vi "main.vi"() -> ()   [LabVIEW 2018]
uses:
  <userlib>/ORI_DataSocketReader/DataSocket Tag Reader.lvclass
  ControlConfigMisura.ctl
  ControlConfigDI.ctl
panel:
  in  "Tab Control":enum32{"Valori", "Storico allarmi"}(tab)
  in  "Misure":i32(listbox)
  in  "fine":timestamp format="%<%Y-%m-%d %H:%M>T"
  in  "Inizio":timestamp format="%<%Y-%m-%d %H:%M>T"
  in  "Storico":i32(listbox)
  out "last":string
  in  "ack":bool
  out "Uscita digitale":bool
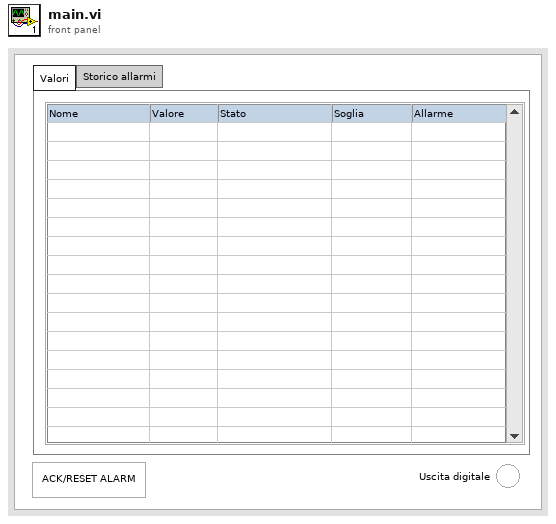
[diagram p1: front panel]
types:
  T1 = typedef "ControlConfigMisura.ctl" = cluster{"svVal":string, "svInvDig":T2[], "nome":string, "valore":dbl, "stato":i16, "soglia":dbl, "allarme":bool, "enable":bool}
  T2 = typedef "ControlConfigDI.ctl" = cluster{"sv":string, "na":bool, "valRaw":bool, "val":bool}
  T3 = typedef "ControlCfg.ctl" = cluster{"misure":T1[], "SVDO":string}
  T4 = typedef "LVPoint32TypeDef.ctl" = cluster{"Horizontal":i32, "Vertical":i32}
  T5 = typedef "LVRowAndColumnTypeDef.ctl" = cluster{"Row":i32, "Column":i32}
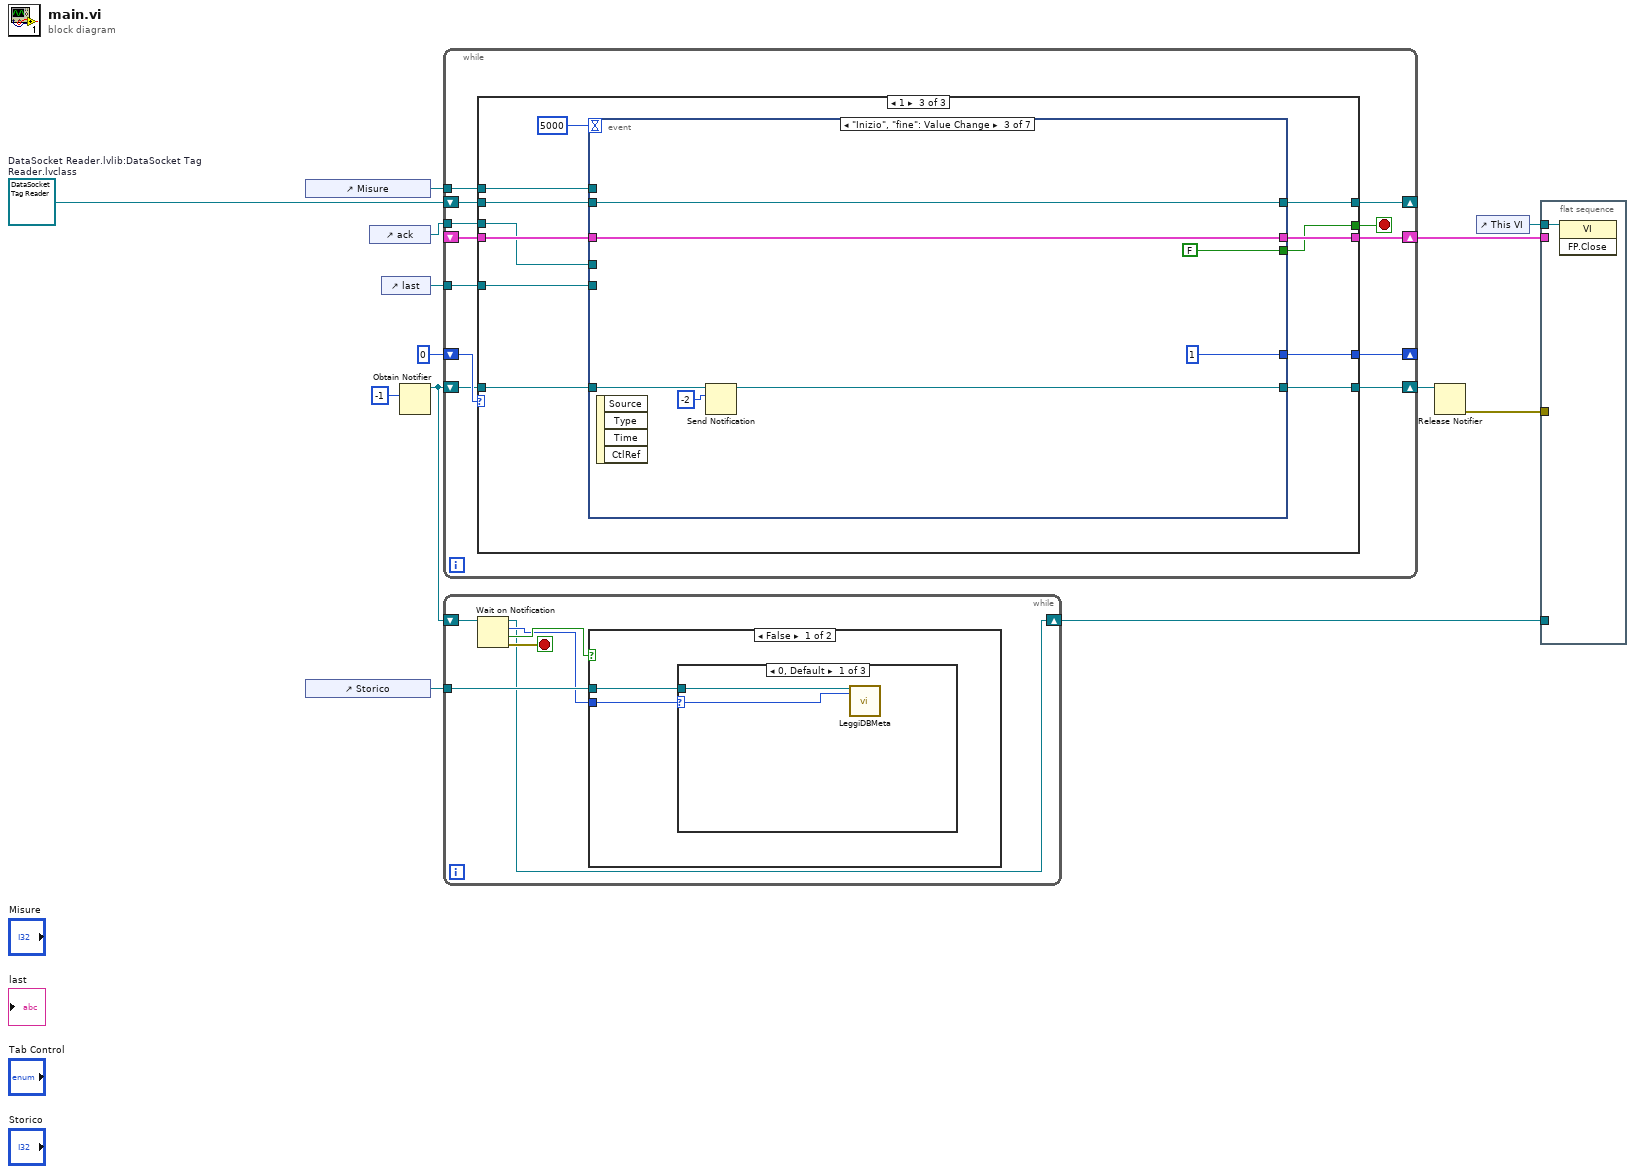
[diagram p0: block diagram]
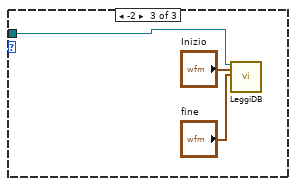
[diagram p3: hidden frame]
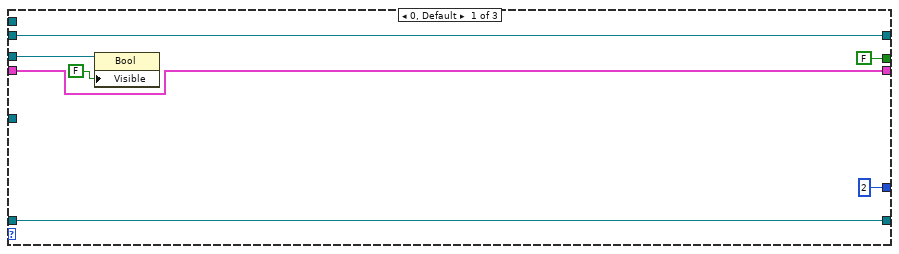
[diagram p5: hidden frame]
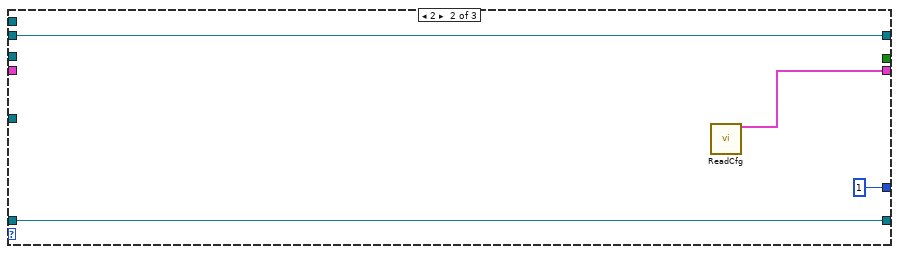
[diagram p6: hidden frame]
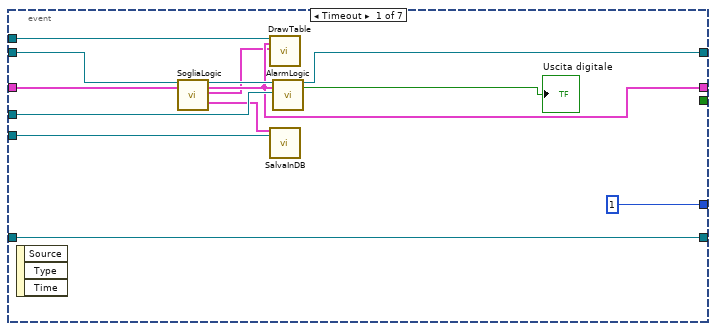
[diagram p7: hidden frame]
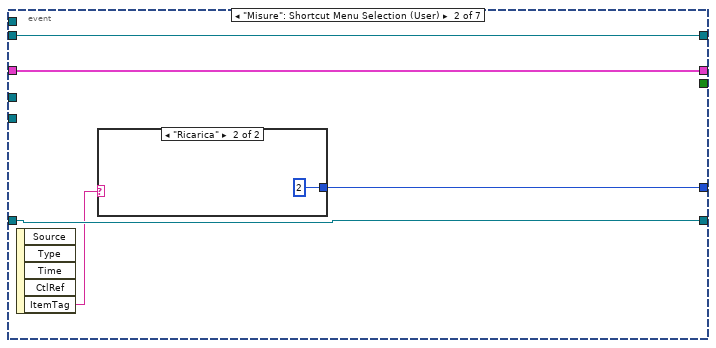
[diagram p8: hidden frame]
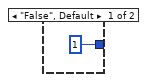
[diagram p9: hidden frame]
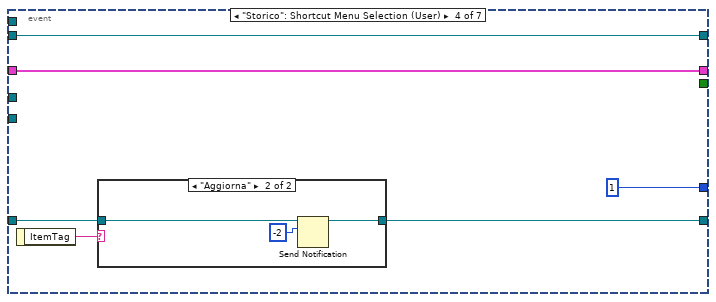
[diagram p10: hidden frame]
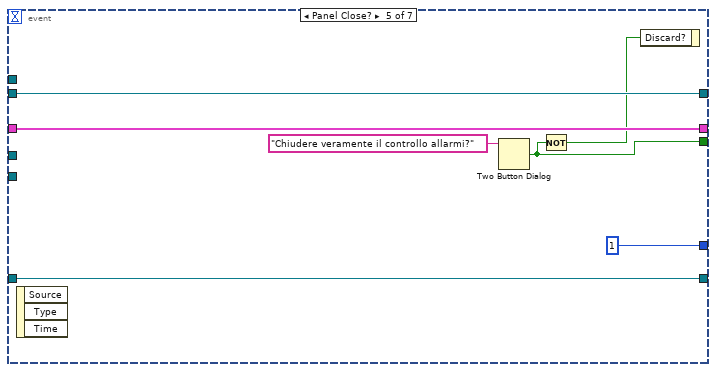
[diagram p12: hidden frame]
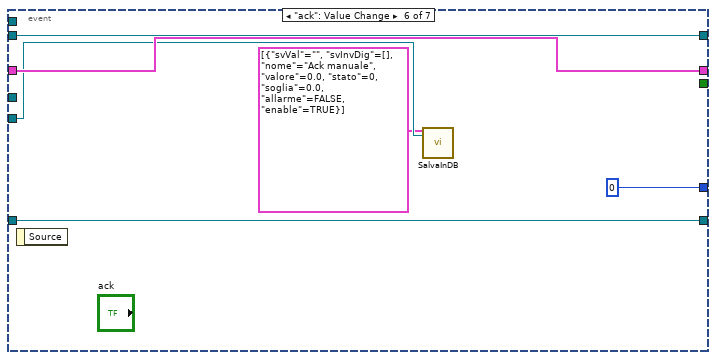
[diagram p13: hidden frame]
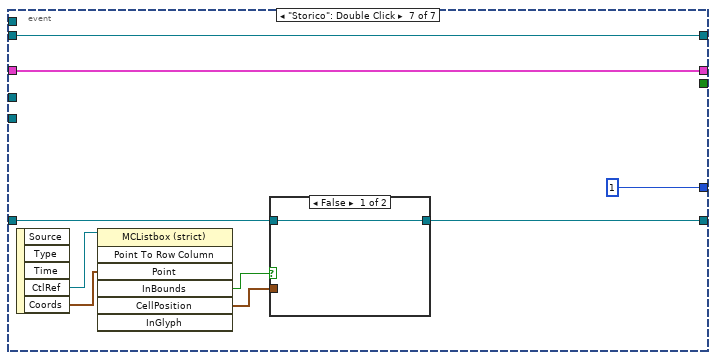
[diagram p14: hidden frame]
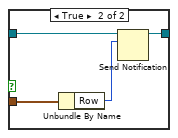
[diagram p15: hidden frame]
diagram:
  w12 = refnum<class "DataSocket Tag Reader.lvclass"> refnum  # DataSocket Reader.lvlib:DataSocket Tag Reader.lvclass
  n1 = control-ref of="Misure"() -> (w11:refnum<vi>)
  n2 = control-ref of="Storico"() -> (w5:refnum<vi>)
  n3 = control-ref of="ack"() -> (w10:refnum<vi>)
  n4 = control-ref of="last"() -> (w7:refnum<vi>)
  n5 = Obtain Notifier(notification data type=-1) -> (notifier out=w6:refnum<notifier>)  [unwired: 3 in, 2 out]
  n6 = while {
    shift-right: [w23] -> _
    shift-left: 0 -> [w25]
    shift-right: [w21] -> _
    shift-left: w12 -> [w22]
    shift-right: [w20] -> w8
    shift-left: _ -> [w19]
    tunnel: w11 -> [w18]
    tunnel: w10 -> [w17]
    tunnel: w7 -> [w16]
    shift-right: [w14] -> w4
    shift-left: w6 -> [w15]
    stop <- w24 stop-if-true
    n7 = case shown="1" w25 {
      tunnel: [FALSE _ w40] -> w24
      tunnel: [2 1 w47] -> w23
      tunnel: w22 -> [w30 w36 w46]
      tunnel: [w30 w36 w45] -> w21
      tunnel: [w26 w34 w43] -> w20
      tunnel: w19 -> [w26 _ w44]
      tunnel: w18 -> [_ _ w42]
      tunnel: w17 -> [w29 _ w41]
      tunnel: w16 -> [_ _ w39]
      tunnel: w15 -> [w28 w35 w38]
      tunnel: [w28 w35 w37] -> w14
      frame 0, Default {
        n8 = property class="Bool"(reference=w29, "Visible"=FALSE) -> ()  [unwired: 1 in, 2 out]
      }
      frame 2 {
        n9 = call "ReadCfg.vi"() -> ("data"=w34:T3)  [unwired: 19 in]
      }
      frame 1 {
        n10 = event shown="[2] \"Inizio\", \"fine\": Value Change" {
          selector: _ -> [_ _ _ _ _ _ _]
          dyn-events: _ -> [_ _ _ _ _ _ _]
          timeout: 5000 -> [_ _ _ _ _ _ _]
          tunnel: [1 w62 1 1 1 0 1] -> w47
          tunnel: w46 -> [w60 w64 w75 w81 w91 w96 w107]
          tunnel: [w55 w64 w75 w81 w91 w96 w107] -> w45
          tunnel: w44 -> [w59 w63 w72 w80 w90 w97 w106]
          tunnel: [w54 w63 w72 w80 w90 w97 w106] -> w43
          tunnel: w42 -> [w58 _ _ _ _ _ _]
          tunnel: w41 -> [w57 _ _ _ _ _ _]
          tunnel: [_ _ FALSE ("T button?") _ w88 _ _] -> w40
          tunnel: w39 -> [w50 _ _ _ _ w94 _]
          tunnel: w38 -> [w49 w66 w71 w77 w86 w95 w104]
          tunnel: [w49 w66 w70 w76 w86 w95 w103] -> w37
          event Timeout {
            n11 = event-data() -> ()  [unwired: 1 in, 3 out]
            n12 = call "SogliaLogic.vi"("DSR"=w60, "cfg"=w59) -> ("DSR out"=w56:refnum<class "DataSocket Tag Reader.lvclass">, "cfg out"=w54:T3, "Array"=w52:cluster{bool[], string[]}[], "CambiStato"=w51:T1[])  [unwired: 14 in]
            n13 = call "DrawTable.vi"("Table"=w58, "cfg"=w54, "Array"=w52) -> ()  [unwired: 17 in]
            n14 = call "SalvaInDB.vi"("CambiStato"=w51, "last"=w50) -> ()  [unwired: 18 in]
            n15 = call "AlarmLogic.vi"("DSR"=w56, "cfg"=w54, "ack"=w57) -> ("DSR out"=w55:refnum<class "DataSocket Tag Reader.lvclass">, "AllarmeSuDO"=→"Uscita digitale":bool)  [unwired: 15 in]
          }
          event "Misure": Shortcut Menu Selection (User) {
            n16 = event-data() -> ("ItemTag"=w65:string)  [unwired: 1 in, 4 out]
            n17 = case shown="\"Ricarica\"" w65 {
              tunnel: [1 2] -> w62
              frame "False", Default {
              }
              frame "Ricarica" {
              }
            }
          }
          event "Inizio", "fine": Value Change {
            n18 = event-data() -> ()  [unwired: 1 in, 4 out]
            n19 = Send Notification(notification=-2, notifier=w71) -> (notifier out=w70:refnum<notifier>)  [unwired: 1 in, 1 out]
          }
          event "Storico": Shortcut Menu Selection (User) {
            n20 = event-data() -> ("ItemTag"=w78:string)  [unwired: 1 in]
            n21 = case shown="\"Aggiorna\"" w78 {
              tunnel: w77 -> [w82 w85]
              tunnel: [w82 w84] -> w76
              frame "False", Default {
              }
              frame "Aggiorna" {
                n22 = Send Notification(notification=-2, notifier=w85) -> (notifier out=w84:refnum<notifier>)  [unwired: 1 in, 1 out]
              }
            }
          }
          event Panel Close? {
            n23 = event-data() -> ()  [unwired: 1 in, 3 out]
            n24 = Two Button Dialog(message="Chiudere veramente il controllo allarmi?") -> (T button?=w88:bool)  [unwired: 2 in]
            n25 = Not(x=w88) -> (.not. x?=w87:bool)
            n26 = event-data("Discard?"=w87) -> ()  [unwired: 1 in, 1 out]
          }
          event "ack": Value Change {
            n27 = event-data() -> ()  [unwired: 1 in, 1 out]
            n28 = call "SalvaInDB.vi"("CambiStato"=T1[] [{"svVal"="", "svInvDig"=[], "nome"="Ack manuale", "valore"=0.0, "stato"=0, "soglia"=0.0, "allarme"=FALSE, "enable"=TRUE}], "last"=w94) -> ()  [unwired: 18 in]
          }
          event "Storico": Double Click {
            n29 = event-data() -> ("CtlRef"=w102:refnum<vi>, "Coords"=w101:T4)  [unwired: 1 in, 3 out]
            n30 = invoke class="MCListbox (strict)" method="Point To Row Column"(reference=w102, "Point"=w101) -> ("InBounds"=w99:bool, "CellPosition"=w100:T5)  [unwired: 5 in, 5 out]
            n31 = case shown="False" w99 {
              tunnel: w104 -> [w108 w112]
              tunnel: [w108 w111] -> w103
              tunnel: w100 -> [_ w110]
              frame False {
              }
              frame True {
                n32 = Unbundle By Name(w110) -> ("Row"=w109:i32)
                n33 = Send Notification(notification=w109, notifier=w112) -> (notifier out=w111:refnum<notifier>)  [unwired: 1 in, 1 out]
              }
            }
          }
        }
      }
    }
  }
  n34 = while {
    shift-right: [w113] -> w2
    shift-left: w6 -> [w117]
    tunnel: w5 -> [w118]
    stop <- w116 stop-if-true
    n35 = Wait on Notification(notifier=w117) -> (notifier out=w113:refnum<notifier>, notification=w114:i32, timed out?=w115:bool, error out=w116:errorcluster)  [unwired: 3 in]
    n36 = case shown="False" w115 {
      tunnel: w118 -> [w120 _]
      tunnel: w114 -> [w119 _]
      frame False {
        n37 = case shown="0, Default" w119 {
          selector: w119 -> [w122 _ _]
          tunnel: w120 -> [w121 _ w123]
          frame 0, Default {
            n38 = call "LeggiDBMeta.vi"("Table"=w121, "raw"=w122) -> ()  [unwired: 18 in]
          }
          frame -1 {
          }
          frame -2 {
            n39 = call "LeggiDB.vi"("Table"=w123, "Inizio"="Inizio", "fine"="fine") -> ()  [unwired: 17 in]
          }
        }
      }
      frame True {
      }
    }
  }
  n40 = Release Notifier(notifier=w4) -> (error out=w3:errorcluster)  [unwired: 2 in, 2 out]
  n41 = control-ref of="This VI"() -> (w9:refnum<vi>)
  n42 = flat-sequence {
    tunnel: w9 -> [w126]
    tunnel: w8 -> [_]
    tunnel: w3 -> [_]
    tunnel: w2 -> [_]
    frame #0 {
      n43 = invoke class="VI" method="FP.Close"(reference=w126) -> ()  [unwired: 2 in, 3 out]
    }
  }
